vi "创建羊对象.vi"() -> (3 "Animal输出":refnum<class "sheep.lvclass">)   [LabVIEW 2020, in "sheep.lvclass"]
uses:
  sheep.lvclass
  Animal/Animal.lvclass/Animal.ctl
  Animal/Animal.lvclass
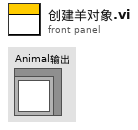
[diagram p1: front panel]
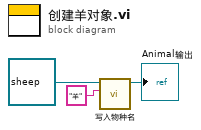
[diagram p0: block diagram]
diagram:
  n1 = call "写入物种名.vi"("物种名"="羊", "Animal输入"=refnum<class "sheep.lvclass"> refnum ("sheep.lvclass")) -> ("Animal输出"=→"Animal输出":refnum<class "sheep.lvclass">)  [unwired: 8 in, 1 out]
